vi "Batch_Order_Generator (SubVI).vi"(11 "Price of Coffee Decimel":dbl) -> (1 "String 2":string, 2 "String 3":string, 3 "String 4":string, 4 "String":string)   [LabVIEW 2019]
uses:
  <vilib>/numeric/Random Number (Range) U64.vi
  <vilib>/numeric/sub_Random U32.vi
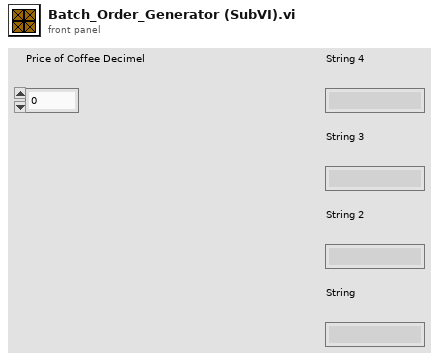
[diagram p1: front panel]
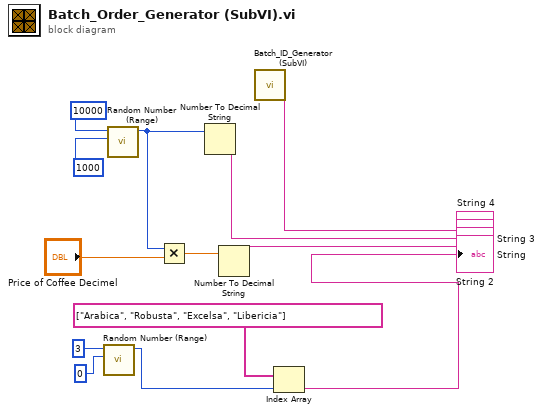
[diagram p0: block diagram]
diagram:
  n1 = call-poly <vilib>:"Random Number (Range).vi"("lower bound (0)"=u64 0, "upper bound (100)"=u64 3) -> ("number"=w12:u64)  [unwired: 9 in]
  n2 = call-poly <vilib>:"Random Number (Range).vi"("lower bound (0)"=u64 1000, "upper bound (100)"=u64 10000) -> ("number"=w4:u64)  [unwired: 9 in]
  n3 = Multiply(x=w4, y="Price of Coffee Decimel") -> (x*y=w7:dbl)
  n4 = Number To Decimal String(number=w4) -> (decimal integer string=→"String 3":string)  [unwired: 1 in]
  n5 = Number To Decimal String(number=w7) -> (decimal integer string=→"String 2":string)  [unwired: 1 in]
  n6 = call "Batch_ID_Generator (SubVI).vi"() -> ("String"=→"String 4":string)  [unwired: 11 in]
  n7 = Index Array(array=string[] ["Arabica", "Robusta", "Excelsa", "Libericia"], index=w12) -> (element=→"String":string)
